vi "Select measurement rate.vi"(8 "error in (no error)":errorcluster, 10 "Rate":T1=enum."Free Run", 11 "VISA resource name":refnum<visa-resource-name>="GPIB0::21::INSTR") -> (0 "error out":errorcluster, 3 "VISA resource name out":refnum<visa-resource-name>)   [LabVIEW 2023, in "Anritsu Power Meter.lvlib"]
uses:
  Anritsu Power Meter.lvlib
  Measuring rate control.ctl
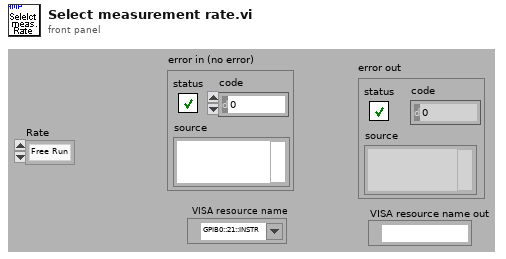
[diagram p1: front panel]
types:
  T1 = typedef "Anritsu Power Meter.lvlib/Measuring rate control.ctl" = enum16{"Hold", "Free Run", "Exit Trigger"}
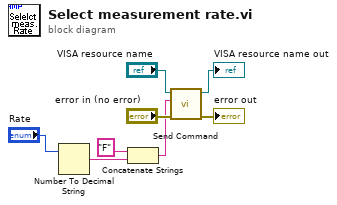
[diagram p0: block diagram]
diagram:
  n1 = Number To Decimal String(number="Rate") -> (decimal integer string=w3:string)  [unwired: 1 in]
  n2 = Concatenate Strings("F" ("string"), w3) -> (w1:string)
  n3 = call "Send Command.vi"("error in (no error)"="error in (no error)", "write buffer"=w1, "VISA resource name"="VISA resource name") -> ("error out"=→"error out":errorcluster, "VISA resource name out"=→"VISA resource name out":refnum<visa-resource-name>)  [unwired: 7 in]
